vi "TimeReversal.vi"() -> ()   [LabVIEW 2014]
panel:
  out "graph of x(-n)":cluster{dbl[], dbl[]}(graph)
  out "graph of x(n)":cluster{i32[], "x(n)":dbl[]}(graph)
  out "mag response of X(-w)":cluster{"-pi to pi":dbl[], dbl[]}(graph)
  out "graph of X(-w)":cluster{"-pi to pi":dbl[], dbl[]}(graph)
  in  "Boolean":bool
  out "x(-n)":dbl[](array[numeric])
  out "X(-w)":cdb[](array[numeric])
  out "mag of X(-w)":dbl[](array[numeric])
  out "graph of mag response":cluster{"-pi to pi":dbl[], dbl[]}(graph)
  out "graph of DTFT{x(-n)}":cluster{"-pi to pi":dbl[], dbl[]}(graph)
  out "DTFT{x(-n)}":cdb[](array[numeric])
  in  "x(n)":dbl[](array[numeric])
  out "mag response":dbl[](array[numeric])
  # "Instructions"
  # "if\nDTFT{x(n)} ----> X(w)\nthen\nDTFT{x(-n)} ----> X(-w)"
  # "1. enter the sequence x(n) as array\n2. check the time reversed sequence of input\n3. verify the property by observing the graph"
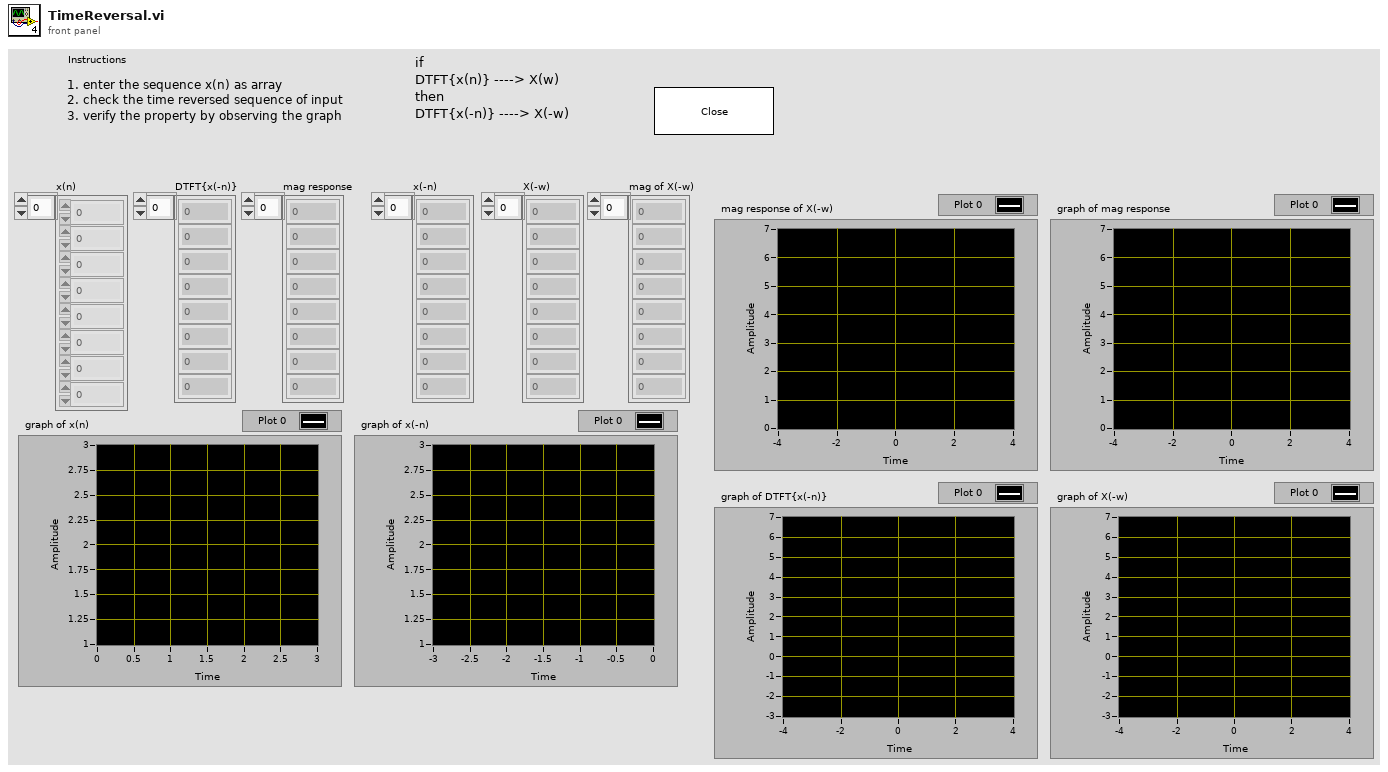
[diagram p1: front panel]
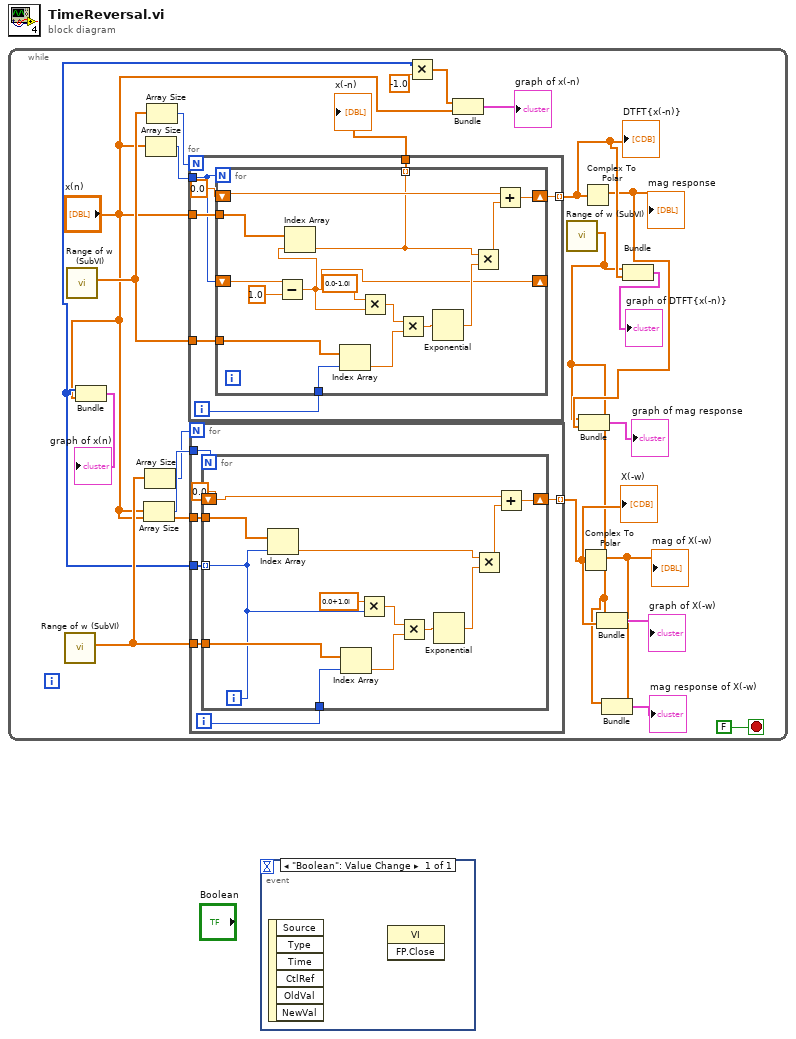
[diagram p0: block diagram]
diagram:
  n1 = while {
    stop <- FALSE stop-if-true
    n2 = call "Range of w (SubVI).vi"() -> ("-pi to pi"=w15:dbl[])  [unwired: 11 in]
    n3 = call "Range of w (SubVI).vi"() -> ("-pi to pi"=w22:dbl[])  [unwired: 11 in]
    n4 = Array Size(array="x(n)") -> (size(s)=w16:i32)
    n5 = Array Size(array=w15) -> (size(s)=w14:i32)
    n6 = Array Size(array="x(n)") -> (size(s)=w23:i32)
    n7 = Array Size(array=w22) -> (size(s)=w21:i32)
    n8 = for {
      N: w21 -> [_]
      tunnel: w22 -> [w49]
      tunnel: w23 -> [w45]
      tunnel: "x(n)" -> [w47]
      tunnel: [w46] -> w20 mode=indexing
      tunnel: [w44] -> w5
      i -> [w50]
      n9 = for {
        N: w45 -> [_]
        tunnel: w50 -> [w64]
        tunnel: w49 -> [w63]
        shift-right: [w57] -> w46
        shift-left: 0.0 -> [w56]
        tunnel: w47 -> [w55]
        shift-right: [w52] -> _
        shift-left: w45 -> [w54]
        tunnel: [w51] -> w44 mode=indexing
        n10 = Subtract(x=w54, y=1.0) -> (x-y=w52:dbl)
        n11 = Index Array(array=w55, index=w52) -> (element=w51:dbl)
        n12 = Index Array(array=w63, index=w64) -> (element=w61:dbl)
        n13 = Multiply(x=cdb 0.0-1.0i, y=w52) -> (x*y=w62:cdb)
        n14 = Multiply(x=w62, y=w61) -> (x*y=w60:cdb)
        n15 = Exponential(1:w60) -> (0:w59:cdb)
        n16 = Multiply(x=w51, y=w59) -> (x*y=w58:cdb)
        n17 = Add(x=w56, y=w58) -> (x+y=w57:cdb)
      }
    }
    "DTFT{x(-n)}" <- w20
    "x(-n)" <- w5
    n18 = for {
      N: w14 -> [_]
      tunnel: w15 -> [w29]
      tunnel: w16 -> [w28]
      tunnel: "x(n)" -> [w26]
      tunnel: [w25] -> w13 mode=indexing
      tunnel: [w24] -> w3
      i -> [w30]
      n19 = for {
        N: w28 -> [_]
        tunnel: w30 -> [w42]
        tunnel: w29 -> [w41]
        shift-right: [w35] -> w25
        shift-left: 0.0 -> [w34]
        tunnel: w26 -> [w32]
        tunnel: [w31] -> w24 mode=indexing
        i -> [w31]
        n20 = Index Array(array=w32, index=w31) -> (element=w33:dbl)
        n21 = Index Array(array=w41, index=w42) -> (element=w39:dbl)
        n22 = Multiply(x=cdb 0.0+1.0i, y=w31) -> (x*y=w40:cdb)
        n23 = Multiply(x=w40, y=w39) -> (x*y=w38:cdb)
        n24 = Exponential(1:w38) -> (0:w37:cdb)
        n25 = Multiply(x=w33, y=w37) -> (x*y=w36:cdb)
        n26 = Add(x=w34, y=w36) -> (x+y=w35:cdb)
      }
    }
    "X(-w)" <- w13
    n27 = Bundle(w3, "x(n)"="x(n)") -> (→"graph of x(n)":cluster{i32[], "x(n)":dbl[]})  [unwired: 1 in]
    n28 = Multiply(x=w3, y=-1.0) -> (x*y=w6:dbl[])
    n29 = Bundle(w6, "x(n)"="x(n)") -> (→"graph of x(-n)":cluster{dbl[], "x(n)":dbl[]})  [unwired: 1 in]
    n30 = call "Range of w (SubVI).vi"() -> ("-pi to pi"=w11:dbl[])  [unwired: 11 in]
    n31 = Complex To Polar(r * e^(i*theta)=w13) -> (r=w10:dbl[])  [unwired: 1 out]
    "mag of X(-w)" <- w10
    n32 = Complex To Polar(r * e^(i*theta)=w20) -> (r=w18:dbl[])  [unwired: 1 out]
    "mag response" <- w18
    n33 = Bundle("-pi to pi"=w11, w18) -> (→"graph of mag response":cluster{"-pi to pi":dbl[], dbl[]})  [unwired: 1 in]
    n34 = Bundle("-pi to pi"=w11, w13) -> (→"graph of X(-w)":cluster{"-pi to pi":dbl[], cdb[]})  [unwired: 1 in]
    n35 = Bundle("-pi to pi"=w11, w10) -> (→"mag response of X(-w)":cluster{"-pi to pi":dbl[], dbl[]})  [unwired: 1 in]
    n36 = Bundle("-pi to pi"=w11, w20) -> (→"graph of DTFT{x(-n)}":cluster{"-pi to pi":dbl[], cdb[]})  [unwired: 1 in]
  }
  n37 = event shown="[0] \"Boolean\": Value Change" {
    selector: _ -> [_]
    dyn-events: _ -> [_]
    timeout: _ -> [_]
    event "Boolean": Value Change {
      n38 = event-data() -> ()  [unwired: 1 in, 6 out]
      n39 = invoke class="VI" method="FP.Close"() -> ()  [unwired: 3 in, 3 out]
    }
  }
